vi "Write data.vi"(8 "error in (no error)":errorcluster, 10 "data":variant, 11 "DoublyNode in":refnum<class "DoublyNode.lvclass">) -> (0 "error out":errorcluster, 3 "DoublyNode out":refnum<class "DoublyNode.lvclass">)   [LabVIEW 2021, in "DoublyNode.lvclass"]
uses:
  DoublyNode.lvclass
  DoublyNode.lvclass/DoublyNode.ctl
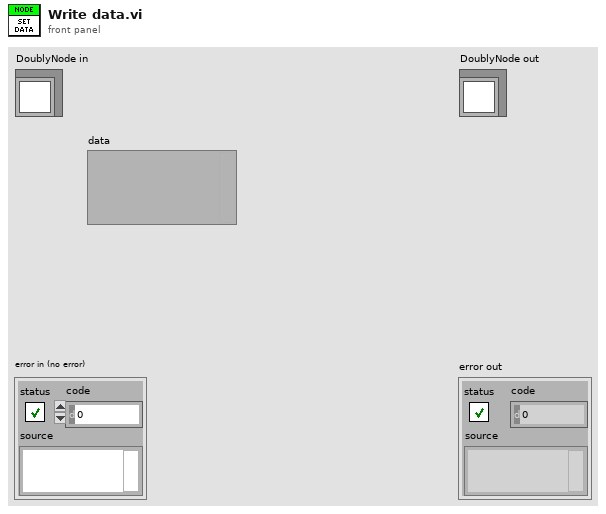
[diagram p1: front panel]
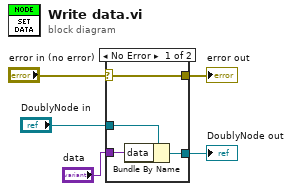
[diagram p0: block diagram]
diagram:
  n1 = case shown="No Error" "error in (no error)" {
    selector: "error in (no error)" -> [w9 w10]
    tunnel: [w9 w10] -> w1
    tunnel: [w7 w11] -> w4
    tunnel: "DoublyNode in" -> [w8 w11]
    tunnel: "data" -> [w6 _]
    frame No Error {
      n2 = Bundle By Name(cluster=w8, "data"=w6) -> (w7:refnum<class "DoublyNode.lvclass">)
    }
    frame Error {
    }
  }
  "error out" <- w1
  "DoublyNode out" <- w4
